vi "calculate golden points.vi"(8 "error in (no error)":errorcluster, 11 "Autofocus in":refnum<class "Autofocus.lvclass">) -> (0 "error out":errorcluster, 1 "point d":dbl, 2 "point c":dbl, 3 "Autofocus out":refnum<class "Autofocus.lvclass">)   [LabVIEW 2012, in "Autofocus.lvclass"]
uses:
  Autofocus.lvclass
  Autofocus.lvclass/Autofocus.ctl
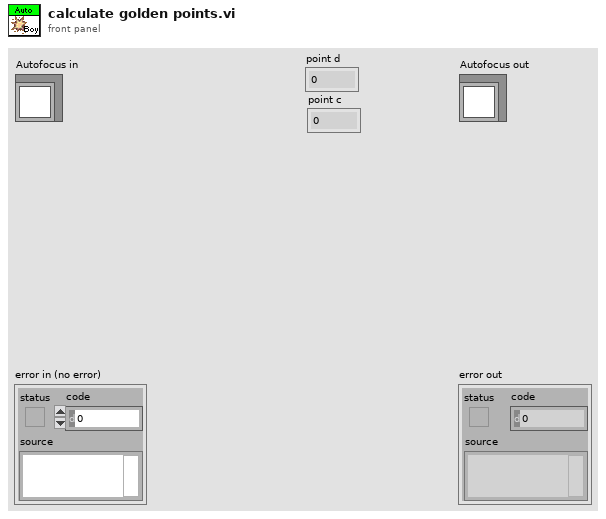
[diagram p1: front panel]
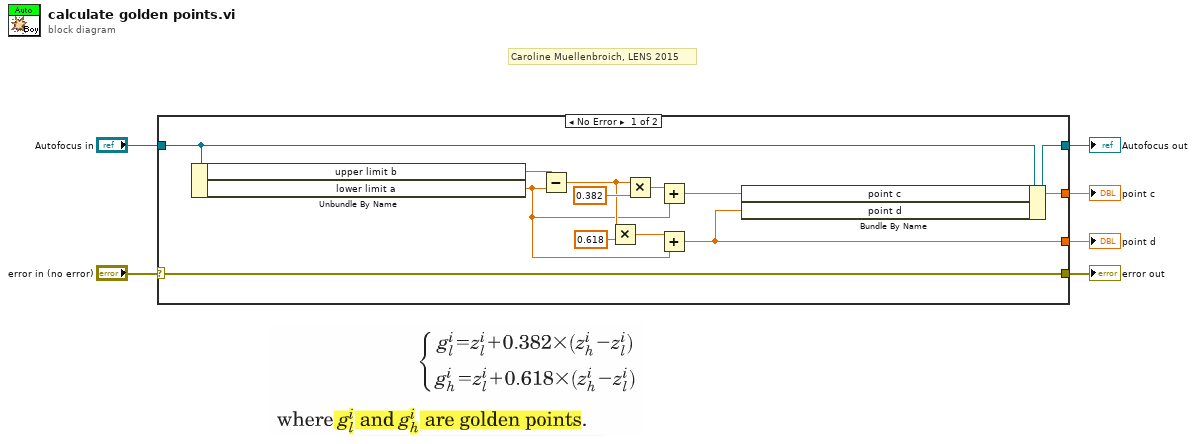
[diagram p0: block diagram]
diagram:
  # "Caroline Muellenbroich, LENS 2015"
  n1 = case shown="No Error" "error in (no error)" {
    selector: "error in (no error)" -> [w18 w20]
    tunnel: [w18 w20] -> w5
    tunnel: [w9 w19] -> w3
    tunnel: "Autofocus in" -> [w10 w19]
    tunnel: [w8 _] -> w2
    tunnel: [w7 _] -> w1
    frame No Error {
      n2 = Unbundle By Name(w10) -> ("upper limit b"=w17:dbl, "lower limit a"=w11:dbl)
      n3 = Subtract(x=w17, y=w11) -> (x-y=w14:dbl)
      n4 = Multiply(x=w14, y=0.618) -> (x*y=w12:dbl)
      n5 = Multiply(x=w14, y=0.382) -> (x*y=w13:dbl)
      n6 = Add(x=w13, y=w11) -> (x+y=w7:dbl)
      n7 = Add(x=w12, y=w11) -> (x+y=w8:dbl)
      n8 = Bundle By Name(cluster=w10, "point c"=w7, "point d"=w8) -> (w9:refnum<class "Autofocus.lvclass">)
    }
    frame Error {
    }
  }
  "error out" <- w5
  "Autofocus out" <- w3
  "point d" <- w2
  "point c" <- w1
